vi "DFD 2-Band Filter Bank Decomposition.vi"   [LabVIEW 2017, in "NI_DigFilter_FilterBank.lvlib"]
doc: "Decomposes a signal into a lowpass band signal and a highpass band signal continuously with a 2-band filter bank."
uses:
  <vilib>/addons/Digital Filter Design/NI_DigFilter_FilterBank.lvlib
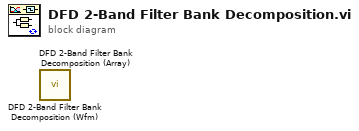
[diagram p0: block diagram]
diagram:
  n1 = call <vilib>:"DFD 2-Band Filter Bank Decomposition (Wfm).vi"() -> ()  [unwired: 9 in, 3 out]
  n2 = call <vilib>:"DFD 2-Band Filter Bank Decomposition (Array).vi"() -> ()  [unwired: 9 in, 3 out]
